vi "Filter Waveforms.vi"(8 "error in (no error)":errorcluster, 10 "Processing Configuration":T1 {"Test Parameters"."Allowed Tolerance (%) FS" format="%#_4g"}, 11 "All Waveforms":waveform(dbl)[](array[waveform])) -> (0 "error out":errorcluster, 2 "Filtered Processing Configuration":T1 {"Test Parameters"."Allowed Tolerance (%) FS" format="%#_4g"}, 3 "UUT Waveforms":waveform(dbl)[](array[waveform]))   [LabVIEW 2026, in "Processing_Engine.lvlib"]
uses:
  Processing_Engine.lvlib
  Processing Settings.ctl
  controls/Messaging Payloads/Sensor CoreData.ctl
  controls/Messaging Payloads/Sensor CoreData Cluster.ctl
  controls/UI/Units Enum.ctl
  controls/UI/Signal Enum.ctl
  Test Parameters.ctl
  Test Parameters Cluster.ctl
  controls/UI/Measurement Role.ctl
  controls/UI/Test Sequence Context.ctl
  controls/UI/Direction.ctl
  Settings/Settings.lvlib
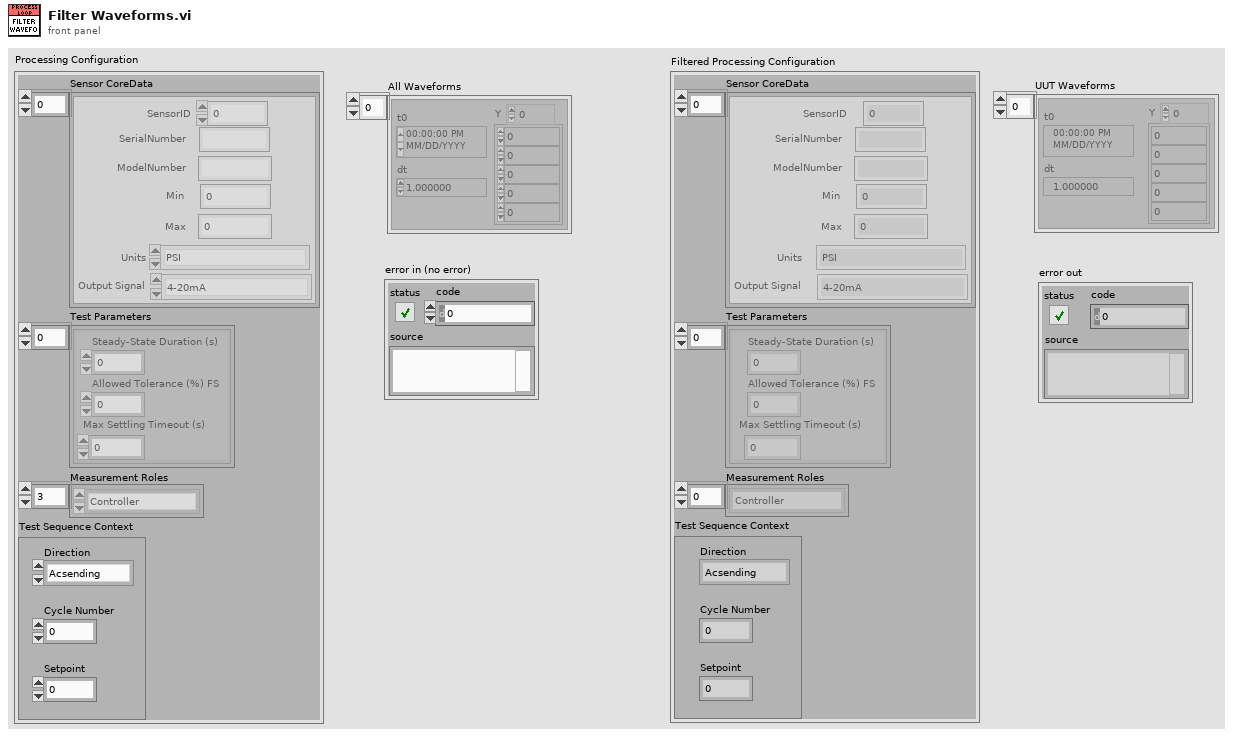
[diagram p1: front panel]
types:
  T1 = typedef "Processing_Engine.lvlib/Processing Settings.ctl" = cluster{"Sensor CoreData":T2, "Test Parameters":T6, "Measurement Roles":T8[], "Test Sequence Context":T9}
  T2 = typedef "Sensor CoreData.ctl" = T3[]
  T3 = typedef "Settings.lvlib/Sensor CoreData Cluster.ctl" = cluster{"SerialNumber":string, "ModelNumber":string, "Min":dbl, "Max":dbl, "Units":T4, "Output Signal":T5, "SensorID":i32}
  T4 = typedef "Units Enum.ctl" = enum16{"PSI", "Deg C", "kPa", "GPM"}
  T5 = typedef "Signal Enum.ctl" = enum16{"4-20mA", "0-10V", "Thermocouple Type K"}
  T6 = typedef "Processing_Engine.lvlib/Test Parameters.ctl" = T7[]
  T7 = typedef "Settings.lvlib/Test Parameters Cluster.ctl" = cluster{"Steady-State Duration (s)":i32, "Allowed Tolerance (%) FS":dbl, "Max Settling Timeout (s)":i32}
  T8 = typedef "Settings.lvlib/Measurement Role.ctl" = enum16{"Controller", "Reference", "UUT"}
  T9 = typedef "Settings.lvlib/Test Sequence Context.ctl" = cluster{"Direction":T10, "Cycle Number":i32, "Setpoint":dbl}
  T10 = typedef "Settings.lvlib/Direction.ctl" = enum16{"Acsending", "Descending"}
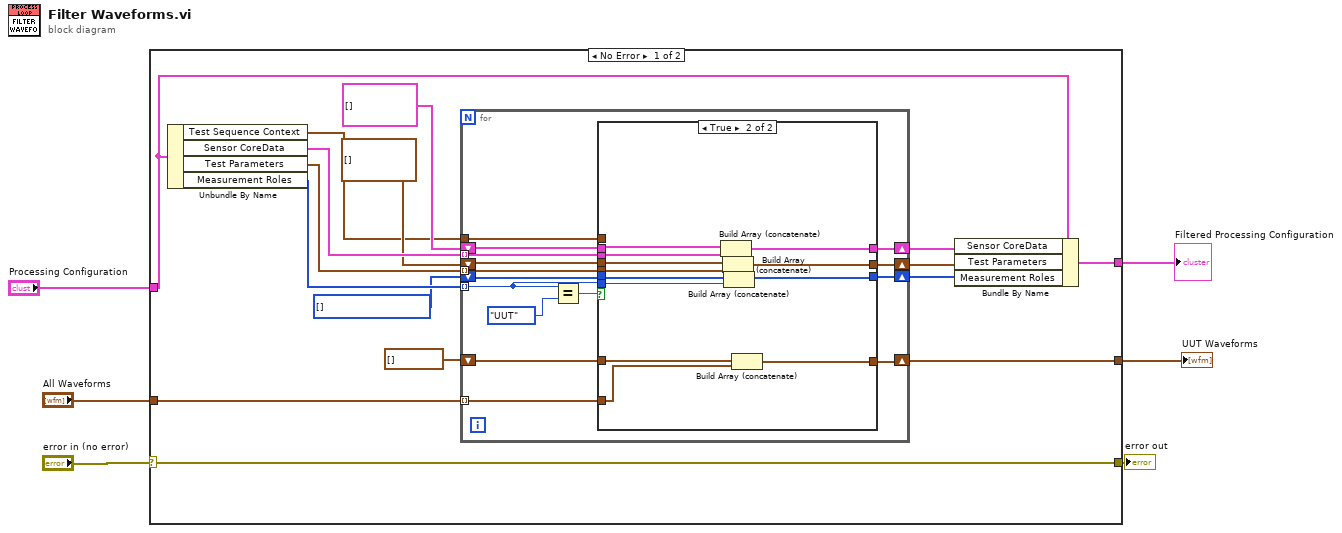
[diagram p0: block diagram]
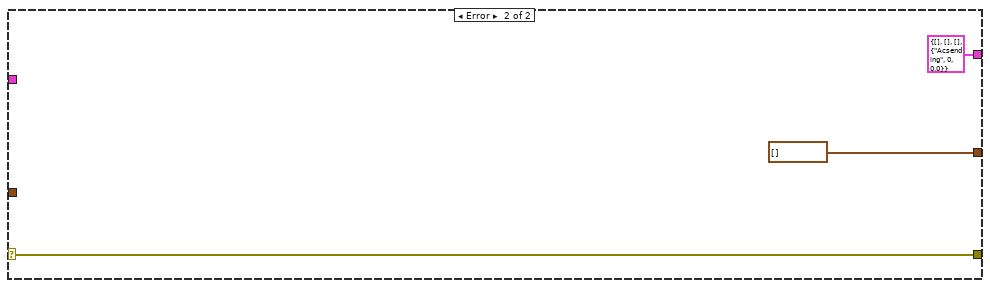
[diagram p3: hidden frame]
diagram:
  n1 = case shown="No Error" "error in (no error)" {
    selector: "error in (no error)" -> [w19 w56]
    tunnel: "Processing Configuration" -> [w13 _]
    tunnel: "All Waveforms" -> [w21 _]
    tunnel: [w20 waveform(dbl)[] []] -> w4
    tunnel: [w19 w56] -> w2
    tunnel: [w9 T1 {"Sensor CoreData"=[], "Test Parameters"=[], "Measurement Roles"=[], "Test Sequence Context"={"Direction"=enum."Acsending", "Cycle Number"=0, "Setpoint"=0.0}} ("Processing Configuration")] -> w1
    frame No Error {
      w7 = T8[] [] items=["Controller", "Reference", "UUT"]
      n2 = Unbundle By Name(w13) -> ("Test Sequence Context"=w8:T9, "Sensor CoreData"=w18:T2, "Test Parameters"=w17:T6, "Measurement Roles"=w22:T8[])
      n3 = for {
        tunnel: w22 -> [w26] mode=indexing
        tunnel: w21 -> [w35] mode=indexing
        shift-right: [w34] -> w20
        shift-left: waveform(dbl)[] [] -> [w33]
        tunnel: w18 -> [w31] mode=indexing
        tunnel: w17 -> [w32] mode=indexing
        shift-right: [w30] -> w12
        shift-left: T2 [] ("Sensor CoreData") -> [w28]
        shift-right: [w29] -> w11
        shift-left: T7[] [] -> [w27]
        shift-right: [w25] -> w10
        shift-left: w7 -> [w24]
        tunnel: w8 -> [w23]
        n4 = Equal?(x=w26, y=Measurement_Role."UUT" ("element")) -> (x = y?=w37:bool)
        n5 = case shown="True" w37 {
          tunnel: w35 -> [_ w53]
          tunnel: [w41 w52] -> w34
          tunnel: w33 -> [w41 w51]
          tunnel: w32 -> [_ w50]
          tunnel: w31 -> [_ w49]
          tunnel: [w40 w48] -> w30
          tunnel: [w39 w47] -> w29
          tunnel: w28 -> [w40 w46]
          tunnel: w27 -> [w39 w45]
          tunnel: w26 -> [_ w44]
          tunnel: [w38 w43] -> w25
          tunnel: w24 -> [w38 w42]
          tunnel: w23 -> [_ _]
          frame False {
          }
          frame True {
            n6 = Build Array (concatenate)(w46, w49) -> (w48:T2)
            n7 = Build Array (concatenate)(w45, w50) -> (w47:T7[])
            n8 = Build Array (concatenate)(w42, w44) -> (w43:T8[])
            n9 = Build Array (concatenate)(w51, w53) -> (w52:waveform(dbl)[])
          }
        }
      }
      n10 = Bundle By Name(cluster=w13, "Sensor CoreData"=w12, "Test Parameters"=w11, "Measurement Roles"=w10) -> (w9:T1)
    }
    frame Error {
    }
  }
  "UUT Waveforms" <- w4
  "error out" <- w2
  "Filtered Processing Configuration" <- w1
